vi "Stop All User Event FGV.vi"(8 "error in":errorcluster, 11 "Action":T1=enum."Fire") -> (0 "error out":errorcluster, 3 "Event ref":refnum<user-event>)   [LabVIEW 2018, in "Common.lvlib"]
uses:
  Common.lvlib
  Stop All - Action.ctl
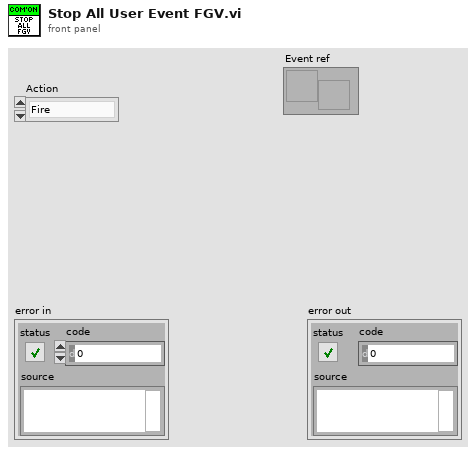
[diagram p1: front panel]
types:
  T1 = typedef "Common.lvlib/Stop All - Action.ctl" = enum16{"Create", "Get", "Fire", "Destroy"}
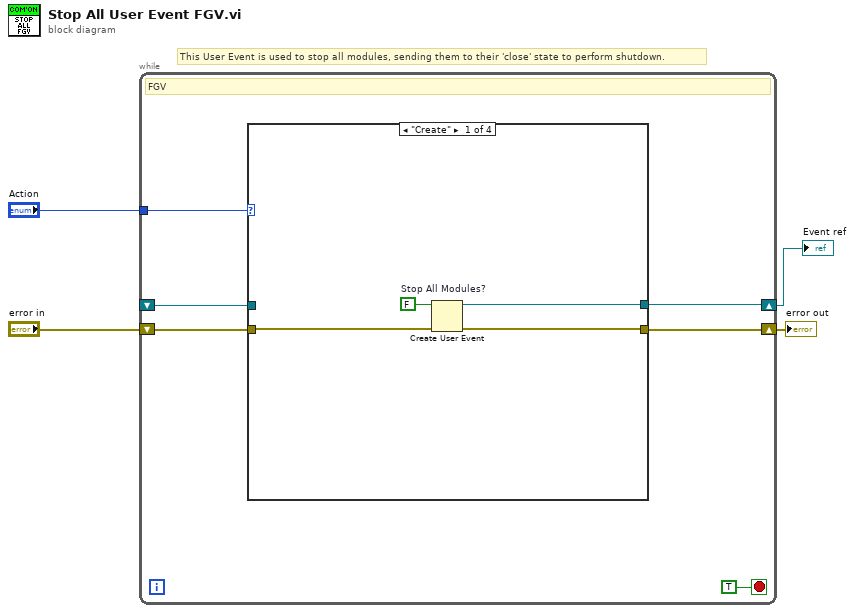
[diagram p0: block diagram]
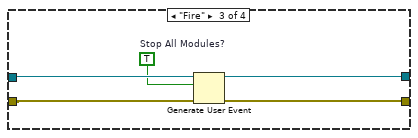
[diagram p3: hidden frame]
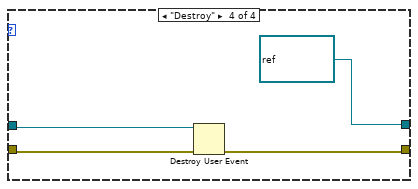
[diagram p4: hidden frame]
diagram:
  # "This User Event is used to stop all modules, sending them to their 'close' state to perform shutdown."
  n1 = while {
    tunnel: "Action" -> [w10]
    shift-right: [w8] -> w4
    shift-left: "error in" -> [w7]
    shift-right: [w5] -> w1
    shift-left: _ -> [w6]
    stop <- TRUE stop-if-true
    # "FGV"
    n2 = case shown="\"Create\"" w10 {
      tunnel: [w13 w16 w20 w24] -> w8
      tunnel: w7 -> [w14 w16 w19 w25]
      tunnel: w6 -> [_ w15 w21 w23]
      tunnel: [w11 w15 w18 refnum<user-event> refnum ("Stop All Modules?")] -> w5
      frame "Create" {
        w12 = FALSE  # Stop All Modules?
        n3 = Create User Event(user event datatype=w12, error in=w14) -> (user event=w11:refnum<user-event>, error out=w13:errorcluster)
      }
      frame "Get", Default {
      }
      frame "Fire" {
        w17 = TRUE  # Stop All Modules?
        n4 = Generate User Event(user event=w21, event data cluster=w17, error in=w19) -> (user event out=w18:refnum<user-event>, error out=w20:errorcluster)  [unwired: 1 in]
      }
      frame "Destroy" {
        n5 = Destroy User Event(user event=w23, error in=w25) -> (error out=w24:errorcluster)
      }
    }
  }
  "error out" <- w4
  "Event ref" <- w1
